vi "DAQ_read_(SubVI).vi"(8 "error in (no error)":errorcluster, 10 "Rate (kHz)":dbl=1.0 format="%0.2f", 11 "physical channels":tag) -> (0 "error out":errorcluster, 3 "data":waveform(dbl))   [LabVIEW 2019]
uses:
  <vilib>/DAQmx/read.llb/DAQmx Read (Analog Wfm 1Chan 1Samp).vi
  <vilib>/DAQmx/create/channels.llb/DAQmx Create Channel (AI-Voltage-Basic).vi
  <vilib>/DAQmx/configure/timing.llb/DAQmx Timing (Sample Clock).vi
  <vilib>/DAQmx/miscellaneous.llb/DAQmx Fill In Error Info.vi
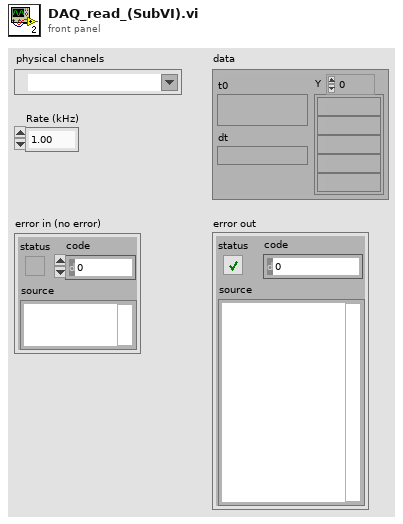
[diagram p1: front panel]
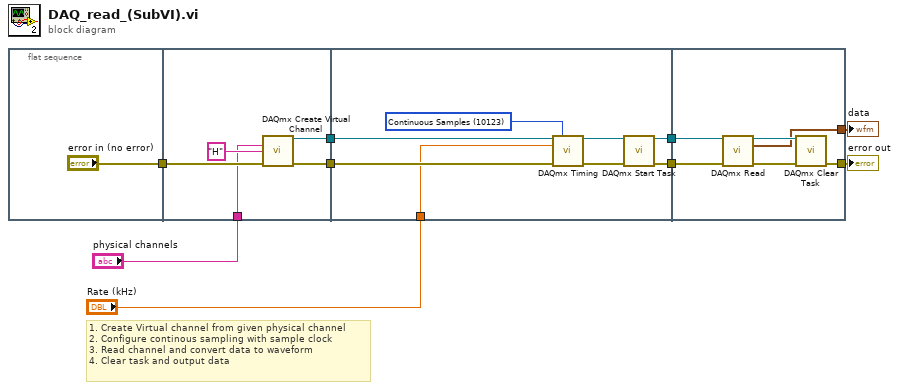
[diagram p0: block diagram]
diagram:
  # "1. Create Virtual channel from given physical channel\n2. Configure continous sampling with sample clock\n3. Read channel and convert data to waveform\n4. Clear task and output data"
  n1 = flat-sequence {
    tunnel: ["error in (no error)"] -> w9
    tunnel: [w15] -> w8
    tunnel: [w14] -> w7
    tunnel: w9 -> [w12]
    tunnel: "physical channels" -> [w11]
    tunnel: w8 -> [w22]
    tunnel: w7 -> [w23]
    tunnel: "Rate (kHz)" -> [w16]
    tunnel: [w19] -> w6
    tunnel: [w18] -> w5
    tunnel: w6 -> [w29]
    tunnel: w5 -> [w28]
    tunnel: [w25] -> w2
    tunnel: [w24] -> w3
    frame #0 {
    }
    frame #1 {
      n2 = call-poly <vilib>:"DAQmx Create Virtual Channel.vi"("physical channels"=w11, "name to assign"="H", "error in"=w12) -> ("task out"=w14:refnum<k21>, "error out"=w15:errorcluster)  [unwired: 11 in]
    }
    frame #2 {
      w17 = 10123 items=["Finite Samples"=10178, "Continuous Samples"=10123, "Hardware Timed Single Point"=12522] ("sample mode")
      n3 = call-poly <vilib>:"DAQmx Timing.vi"("task/channels in"=w23, "sample mode"=w17, "rate"=w16, "error in"=w22) -> ("task out"=w21:refnum<k21>, "error out"=w20:errorcluster)  [unwired: 10 in]
      n4 = call <vilib>:"DAQmx Start Task.vi"("task/channels in"=w21, "error in"=w20) -> ("task out"=w18:refnum<k21>, "error out"=w19:errorcluster)  [unwired: 12 in]
    }
    frame #3 {
      n5 = call-poly <vilib>:"DAQmx Read.vi"("task/channels in"=w28, "error in"=w29) -> ("task out"=w27:refnum<k21>, "data"=w24:waveform(dbl), "error out"=w26:errorcluster)  [unwired: 11 in]
      n6 = call <vilib>:"DAQmx Clear Task.vi"("task in"=w27, "error in"=w26) -> ("error out"=w25:errorcluster)  [unwired: 13 in]
    }
  }
  "error out" <- w2
  "data" <- w3
